vi "main.vi"() -> ()   [LabVIEW 2023]
panel:
  in  "stop":bool
  in  "Tab Control":enum32{"Page 1", "Page 2"}(tab)
  in  "Watch Table":i32[](listbox)
  in  "Selected Watch Table":i32(listbox)
  in  "Remove Item":bool
  in  "Add Item":bool
  in  "Ring":u16(ring) items=["a", "b", "c", "d", "f", "e", "g", "h", "j", "k", "l", "m", "n", "o"]
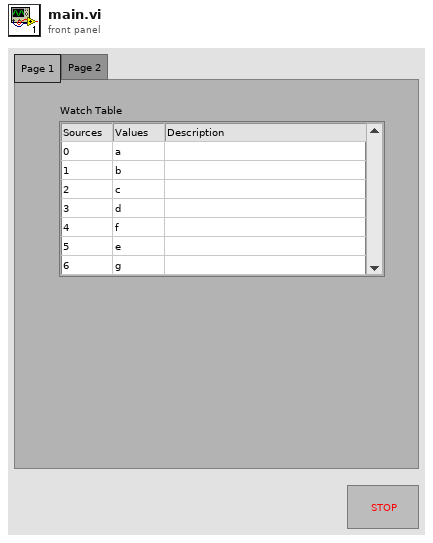
[diagram p1: front panel]
types:
  T1 = typedef "LVRowAndColumnTypeDef.ctl" = cluster{"Row":i32, "Column":i32}
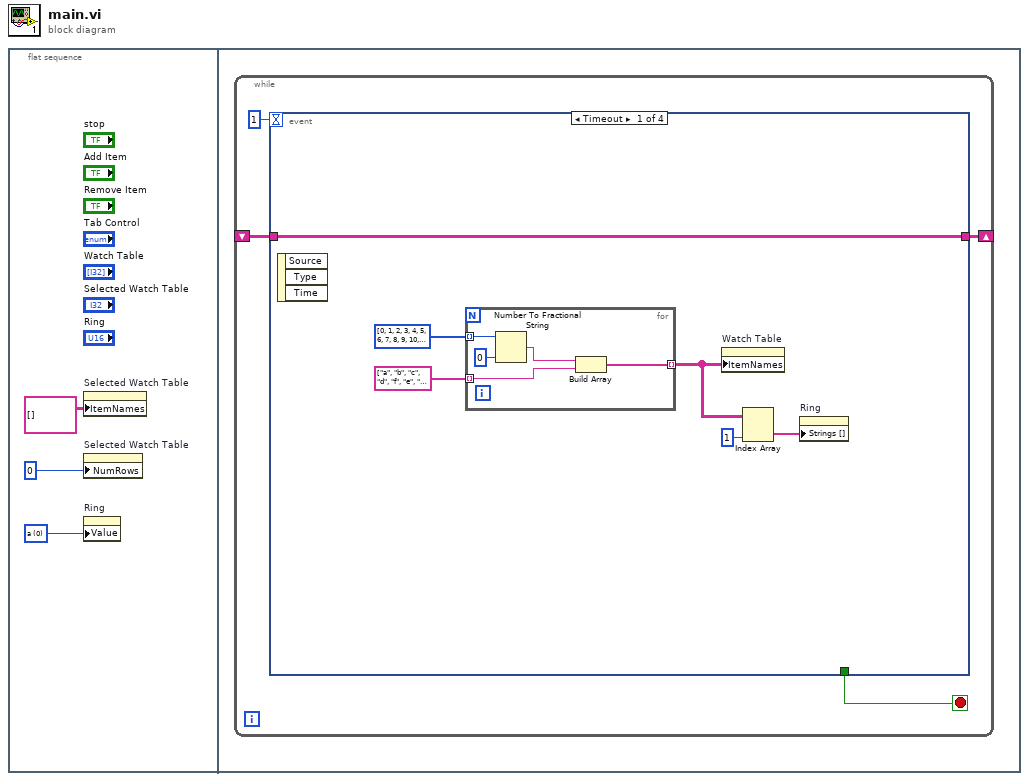
[diagram p0: block diagram]
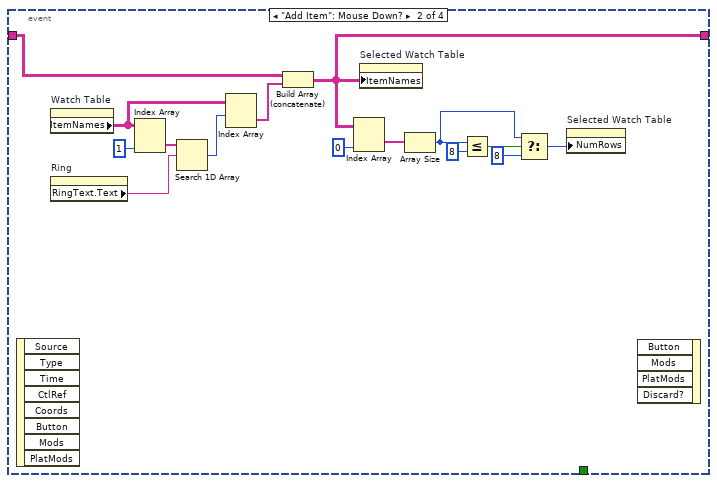
[diagram p2: hidden frame]
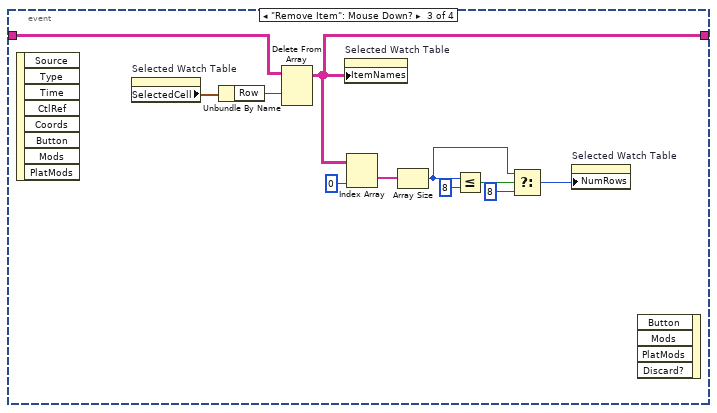
[diagram p3: hidden frame]
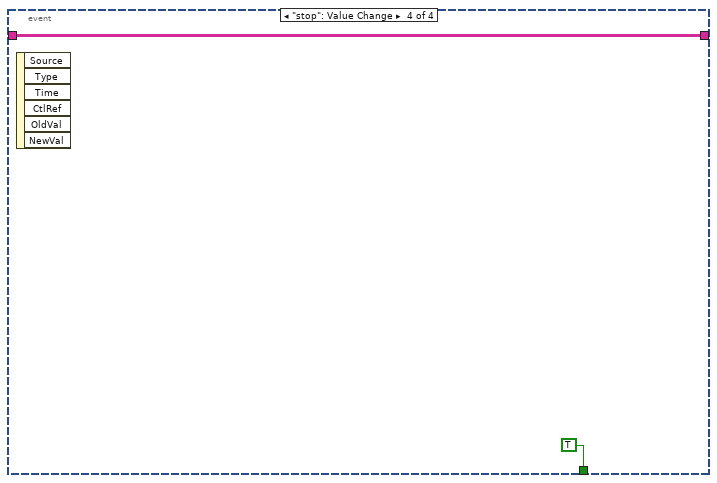
[diagram p4: hidden frame]
diagram:
  n1 = flat-sequence {
    frame #0 {
      w1 = u16 0 items=["a", "b", "c", "d", "f", "e", "g", "h", "j", "k", "l", "m", "n", "o"] ("Ring")
      n2 = property on="Selected Watch Table" class="MCListbox (strict)"("ItemNames"=string[][] [] ("Item Names")) -> ()  [unwired: 2 in, 2 out]
      n3 = property on="Selected Watch Table" class="MCListbox (strict)"("NumRows"=u32 0 ("Number of Rows")) -> ()  [unwired: 2 in, 2 out]
      n4 = property on="Ring" class="Ring (strict)"("Value"=w1) -> ()  [unwired: 2 in, 2 out]
    }
    frame #1 {
      n5 = while {
        shift-right: [w4] -> _
        shift-left: _ -> [w5]
        stop <- w7 stop-if-true
        n6 = event shown="[0] Timeout" {
          selector: _ -> [_ _ _ _]
          dyn-events: _ -> [_ _ _ _]
          timeout: 1 -> [_ _ _ _]
          tunnel: [_ _ _ TRUE] -> w7
          tunnel: w5 -> [w8 w20 w42 w45]
          tunnel: [w8 w19 w35 w45] -> w4
          event Timeout {
            n7 = event-data() -> ()  [unwired: 1 in, 3 out]
            n8 = for {
              tunnel: i32[] [0, 1, 2, 3, 4, 5, 6, 7, 8, 9, 10, 11, 12, 13] -> [w18] mode=indexing
              tunnel: string[] ["a", "b", "c", "d", "f", "e", "g", "h", "j", "k", "l", "m", "n", "o"] -> [w16] mode=indexing
              tunnel: [w15] -> w9 mode=indexing
              n9 = Number To Fractional String(number=w18, precision (6)=i16 0) -> (F-format string=w17:string)  [unwired: 2 in]
              n10 = Build Array(w17, w16) -> (w15:string[])
            }
            n11 = property on="Watch Table" class="MCListbox (strict)"("ItemNames"=w9) -> ()  [unwired: 2 in, 2 out]
            n12 = Index Array(array=w9, index (col)=1 ("disabled index (col)")) -> (element=w11:string[])  [unwired: 1 in]
            n13 = property on="Ring" class="Ring (strict)"("Strings []"=w11) -> ()  [unwired: 2 in, 2 out]
          }
          event "Add Item": Mouse Down? {
            n14 = event-data() -> ()  [unwired: 1 in, 8 out]
            n15 = property on="Watch Table" class="MCListbox (strict)"() -> ("ItemNames"=w30:string[][])  [unwired: 2 in, 2 out]
            n16 = property on="Ring" class="Ring (strict)"() -> ("RingText.Text"=w31:string)  [unwired: 2 in, 2 out]
            n17 = Index Array(array=w30, index (col)=1 ("disabled index (col)")) -> (element=w32:string[])  [unwired: 1 in]
            n18 = Search 1D Array(1D array=w32, element=w31) -> (index of element=w29:i32)  [unwired: 1 in]
            n19 = Index Array(array=w30, index (row)=w29) -> (element=w28:string[])  [unwired: 1 in]
            n20 = Build Array (concatenate)(w20, w28) -> (w19:string[][])
            n21 = Index Array(array=w19, index (col)=0 ("disabled index (col)")) -> (element=w26:string[])  [unwired: 1 in]
            n22 = property on="Selected Watch Table" class="MCListbox (strict)"("ItemNames"=w19) -> ()  [unwired: 2 in, 2 out]
            n23 = Array Size(array=w26) -> (size(s)=w23:i32)
            n24 = Less Or Equal?(x=w23, y=8) -> (x <= y?=w24:bool)
            n25 = Select(t=w23, s=w24, f=8) -> (s? t:f=w21:i32)
            n26 = property on="Selected Watch Table" class="MCListbox (strict)"("NumRows"=w21) -> ()  [unwired: 2 in, 2 out]
            n27 = event-data() -> ()  [unwired: 5 in, 1 out]
          }
          event "Remove Item": Mouse Down? {
            n28 = event-data() -> ()  [unwired: 1 in, 8 out]
            n29 = property on="Selected Watch Table" class="MCListbox (strict)"() -> ("SelectedCell"=w44:T1)  [unwired: 2 in, 2 out]
            n30 = Unbundle By Name(w44) -> ("Row"=w43:i32)
            n31 = Delete From Array(array=w42, index (row)=w43) -> (array with subset deleted=w35:string[][])  [unwired: 2 in, 1 out]
            n32 = property on="Selected Watch Table" class="MCListbox (strict)"("ItemNames"=w35) -> ()  [unwired: 2 in, 2 out]
            n33 = Index Array(array=w35, index (col)=0 ("disabled index (col)")) -> (element=w40:string[])  [unwired: 1 in]
            n34 = Array Size(array=w40) -> (size(s)=w37:i32)
            n35 = Less Or Equal?(x=w37, y=8) -> (x <= y?=w38:bool)
            n36 = Select(t=w37, s=w38, f=8) -> (s? t:f=w34:i32)
            n37 = property on="Selected Watch Table" class="MCListbox (strict)"("NumRows"=w34) -> ()  [unwired: 2 in, 2 out]
            n38 = event-data() -> ()  [unwired: 5 in, 1 out]
          }
          event "stop": Value Change {
            n39 = event-data() -> ()  [unwired: 1 in, 6 out]
          }
        }
      }
    }
  }
